vi "Reload Symbol Infomation Collection.vi"(8 "error in (no error)":errorcluster, 11 "TwinCAT ADS in":refnum<class "TwinCAT ADS.lvclass">) -> (0 "error out":errorcluster, 3 "TwinCAT ADS out":refnum<class "TwinCAT ADS.lvclass">)   [LabVIEW 2018, in "TwinCAT ADS.lvclass"]
uses:
  TwinCAT ADS.lvclass
  TwinCAT ADS.lvclass/TwinCAT ADS.ctl
  TwinCAT.Ads
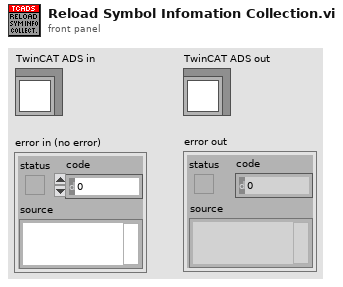
[diagram p1: front panel]
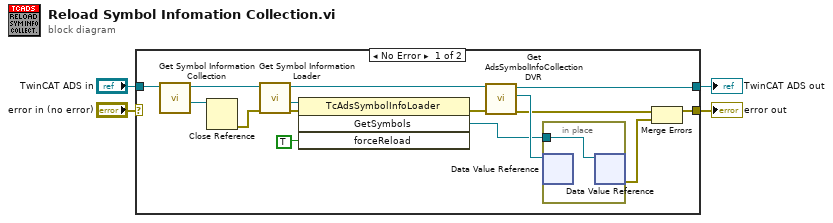
[diagram p0: block diagram]
diagram:
  n1 = case shown="No Error" "error in (no error)" {
    selector: "error in (no error)" -> [_ w22]
    tunnel: [w6 w22] -> w3
    tunnel: [w5 w21] -> w1
    tunnel: "TwinCAT ADS in" -> [w16 w21]
    frame No Error {
      n2 = call "Get Symbol Information Collection.vi"("TwinCAT ADS in"=w16) -> (".NET AdsSymbolInfoCollection"=w15:refnum<k24>, "TwinCAT ADS out"=w13:refnum<class "TwinCAT ADS.lvclass">)  [unwired: 8 in, 1 out]
      n3 = Close Reference(reference=w15) -> (error out=w14:errorcluster)  [unwired: 1 in]
      n4 = call "Get Symbol Information Loader.vi"("error in (no error)"=w14, "TwinCAT ADS in"=w13) -> ("error out"=w17:errorcluster, ".NET AdsSymbolInfoLoader"=w18:refnum<k24>, "TwinCAT ADS out"=w12:refnum<class "TwinCAT ADS.lvclass">)  [unwired: 7 in]
      n5 = invoke class="TcAdsSymbolInfoLoader" method="GetSymbols"(reference=w18, error in=w17, "forceReload"=TRUE) -> (error out=w11:errorcluster, "GetSymbols"=w9:refnum<k24>)  [unwired: 1 in, 2 out]
      n6 = call "Get AdsSymbolInfoCollection DVR.vi"("error in (no error)"=w11, "TwinCAT ADS in"=w12) -> ("error out"=w7:errorcluster, "AdsSymbolInfoCollection DVR"=w10:refnum<data-value>, "TwinCAT ADS out"=w5:refnum<class "TwinCAT ADS.lvclass">)  [unwired: 7 in]
      n7 = in-place {
        in-place-border: w9 -> [w20]
        n8 = in-place-dvr #1(w10) -> ()  [unwired: 2 out]
        n9 = in-place-dvr #1(w20) -> (w8:errorcluster)  [unwired: 1 out]
      }
      n10 = Merge Errors(w7, w8) -> (w6:errorcluster)
    }
    frame Error {
    }
  }
  "error out" <- w3
  "TwinCAT ADS out" <- w1
